vi "criteria_initialize.vi"(8 "error in (no error)":errorcluster, 10 "recipe_data":variant, 11 "criteria":variant) -> (0 "error out":errorcluster)   [LabVIEW 2015, in "lv-recipe-machine.lvlib" / "example_01.lvlib"]
doc: "criteria_initialize.vi will decode the criteria to determine how to initialize the recipe_data and communicate that to the recipe machine."
uses:
  example_01.lvlib
  _controls/recipes.ctl
  lv-recipe-machine.lvlib
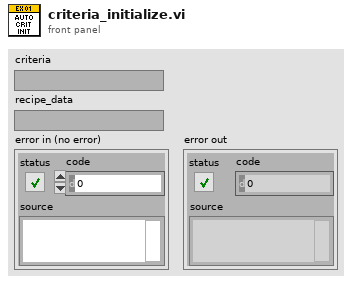
[diagram p1: front panel]
types:
  T1 = typedef "lv-recipe-machine.lvlib/example_01.lvlib/recipes.ctl" = enum16{"<recipes>", "wait_random", "random_wait", "count", "comparison", "launch", "<null>"}
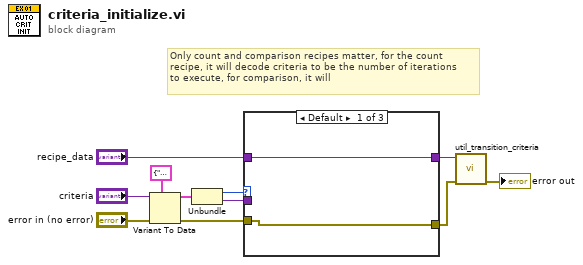
[diagram p0: block diagram]
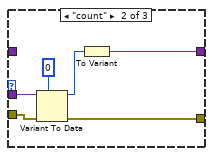
[diagram p2: hidden frame]
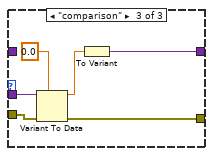
[diagram p3: hidden frame]
diagram:
  # "Only count and comparison recipes matter, for the count\nrecipe, it will decode criteria to be the number of iterations\nto execute, for comparison, it will"
  n1 = Variant To Data(error in="error in (no error)", type=cluster{"recipe":T1, variant} {"recipe"=enum."<recipes>", variant}, Variant="criteria") -> (data=w7:cluster{"recipe":T1, variant}, error out=w4:errorcluster)
  n2 = Unbundle(w7) -> ("recipe"=w6:T1, w5:variant)
  n3 = case shown="Default" w6 {
    tunnel: w5 -> [_ w14 w23]
    tunnel: w4 -> [w12 w19 w24]
    tunnel: "recipe_data" -> [w13 _ _]
    tunnel: [w13 w16 w25] -> w2
    tunnel: [w12 w15 w22] -> w1
    frame Default {
    }
    frame "count" {
      n4 = Variant To Data(error in=w19, type=0, Variant=w14) -> (data=w17:i32, error out=w15:errorcluster)
      n5 = To Variant(anything=w17) -> (Variant=w16:variant)
    }
    frame "comparison" {
      n6 = Variant To Data(error in=w24, type=0.0, Variant=w23) -> (data=w20:dbl, error out=w22:errorcluster)
      n7 = To Variant(anything=w20) -> (Variant=w25:variant)
    }
  }
  n8 = call "util_transition_criteria.vi"("error in (no error)"=w1, "recipe_data"=w2) -> ("error out"=→"error out":errorcluster)  [unwired: 9 in]
